vi "PicoScope2000ExampleStreaming.vi"() -> ()   [LabVIEW 2010]
doc: "This example demonstrates how to use the PicoScope Labview library to stream data from a PicoScope 2000 Series Device"
uses:
  PicoScope2000Lib/PicoScope2000AnalogChannelSettings.ctl
panel:
  in  "Write to file":bool
  in  "Trigger Settings":T1={"Trigger Enabled"=FALSE, "Trigger Source"=enum."Channel A", "Trigger Threshold (V)"=0.0, "Trigger Direction"=0, "Trigger Delay (%)"=-50, "Auto Trigger Time (ms)"=1000} {"Trigger Direction" items=["Rising", "Falling"]; "Trigger Threshold (V)" format="%.3p"}
  out "overflow":i16 format="%02b"
  out "Unit Info":T2
  out "Channels App Buffer":cluster{i32, dbl, "Channel B Buffer":i16[]}[](graph)
  in  "AutoStop App Buffer":bool
  in  "Channel A Settings":T3={"Enabled"=TRUE, "Coupling"=1, "Range"=6} {"Range" items=["20 mV"=1, "50 mV"=2, "100 mV"=3, "200 mV"=4, "500 mV"=5, "1 V"=6, "2 V"=7, "5 V"=8, "10 V"=9, "20 V"=10]; "Coupling" items=["AC", "DC"]}
  in  "Channel B Settings":T3={"Enabled"=TRUE, "Coupling"=1, "Range"=6} {"Range" items=["20 mV"=1, "50 mV"=2, "100 mV"=3, "200 mV"=4, "500 mV"=5, "1 V"=6, "2 V"=7, "5 V"=8, "10 V"=9, "20 V"=10]; "Coupling" items=["AC", "DC"]}
  out "Application Buffer Full":bool
  in  "Acquisition Settings":T4={"Auto Stop"=FALSE, "Desired Sample Interval"=2, "Max Samples"=333000, "Num Samples per Aggregate"=1, "Overview Buffer Size"=1000000, "Time Units"=3, "Application Buffer Size"=0} {"Time Units" items=["Nanoseconds (ns)"=2, "Microseconds (us)"=3, "Milliseconds (ms)"=4, "Seconds (s)"=5]; "Overview Buffer Size" format="%#.5p"; "Max Samples" format="%#.5p"}
  out "Analog Channels":T5(graph)
  out "Raw Sample Interval (sec)":dbl format="%#.5p"
  out "Chunk time":u32
  out "Elapsed time":dbl
  in  "Data file":path=path "PicoScope2000ExampleStreaming Data"
  out "Queue depth ChA":i32(graph)
  out "queue depth":i32
  in  "Buffer and Transfer Settings":T6={"startIndex"=0, "Samples"=1500000, "Down Sample Ratio"=1, "Down-Sample Mode"=0} {"Down-Sample Mode" items=["None"=0, "Aggregate"=1, "Decimate"=2, "Average"=4]; "Down Sample Ratio" step=1; "Samples" format="%#_5p"}
  out "TriggeredAt (In Buffer)":u32 format="%#.6p"
  out "TriggeredAt (Total samples)":u32 format="%#.6p"
  out "Triggered":bool
  out "DownSample Interval (sec)":dbl format="%#.5p"
  out "Total Samples":u32 format="%#.6p"
  out "Auto Stopped":bool
  out "Number of Samples per Capture":u32 format="%#.6p"
  in  "Apply  Settings":bool
  in  "stop":bool
  # "Max. Recommended Settings\nSettings for 1 channels\nSample Interval 1 us\n\nSettings for 2 channels\nSample Interval 2 us\n\nRecommended Settings-\nMax. Samples 333k\nOverview Buffer 1M\n\nBuffer and Transfer Settings-\nSamples- 1.5M (as min.)\n(Buffer = x1.5 (min) Overview buffer)"
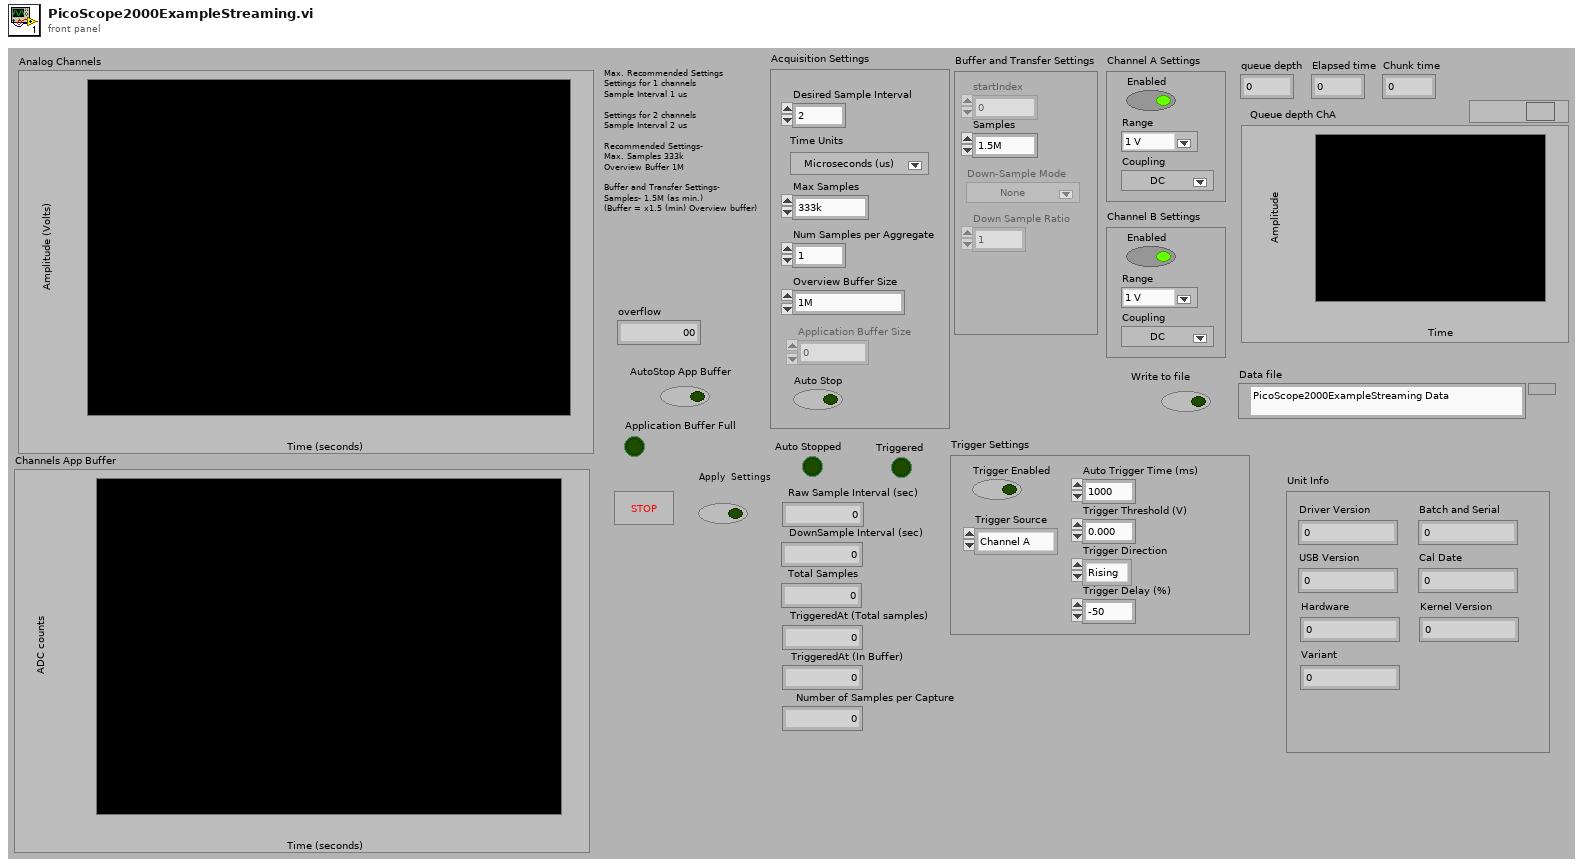
[diagram p1: front panel]
types:
  T1 = cluster{"Trigger Enabled":bool, "Trigger Source":enum16{"Channel A", "Channel B"}, "Trigger Threshold (V)":dbl, "Trigger Direction":i16, "Trigger Delay (%)":i16, "Auto Trigger Time (ms)":i16}
  T2 = cluster{"Driver Version":string, "USB Version":string, "Hardware":string, "Variant":string, "Batch and Serial":string, "Cal Date":string, "Kernel Version":string}
  T3 = typedef "PicoScope2000AnalogChannelSettings.ctl" = cluster{"Enabled":bool, "Coupling":i16, "Range":u16}
  T4 = cluster{"Auto Stop":bool, "Desired Sample Interval":u32, "Max Samples":u32, "Num Samples per Aggregate":u32, "Overview Buffer Size":u32, "Time Units":u32, "Application Buffer Size":u32}
  T5 = cluster{i32, "DownSample Interval (sec)":dbl, "Data":dbl[]}[]
  T6 = cluster{"startIndex":u64, "Samples":u64, "Down Sample Ratio":u64, "Down-Sample Mode":u32}
  T7 = enum16{"open", "open or create", "create or replace", "create", "open (read-only)"}
  T8 = cluster{"Channel A Buffer":i16[], "Channel B Buffer":i16[], "Channel C Buffer":i16[], "Channel D Buffer":i16[], "Channel E Buffer":i16[], "Channel F Buffer":i16[], "Channel G Buffer":i16[], "Channel H Buffer":i16[], "Port 0":i16[], "Port 1":i16[]}
  T9 = cluster{i32, "DownSample Interval (sec)":dbl, "Data":dbl[]}
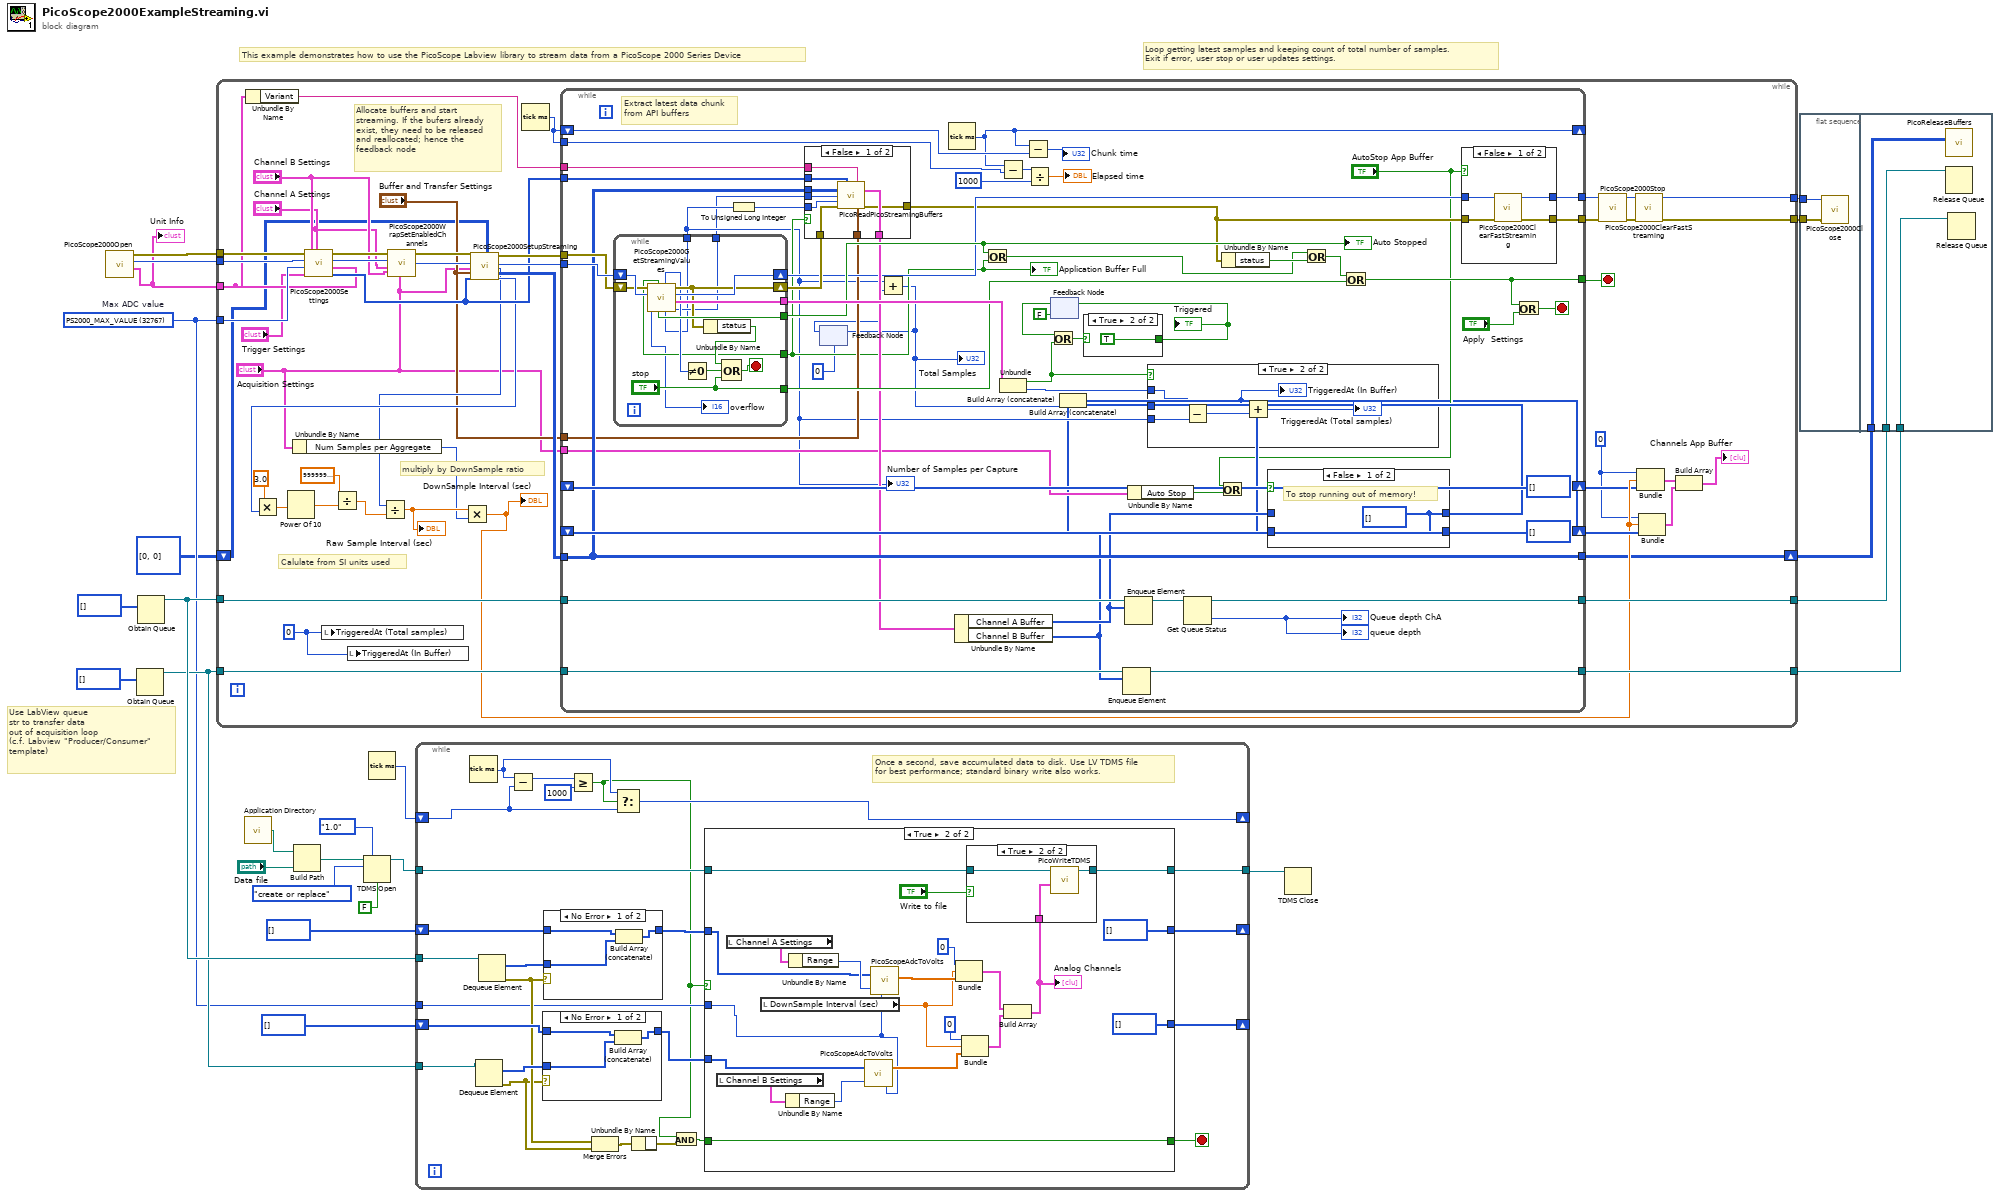
[diagram p0: block diagram]
diagram:
  w4 = i16 32767 items=["PS2000_MAX_VALUE"=32767]  # Max ADC value
  # "Loop getting latest samples and keeping count of total number of samples. \nExit if error, user stop or user updates settings."
  # "Use LabView queue\nstr to transfer data\nout of acquisition loop\n(c.f. Labview \"Producer/Consumer\"\ntemplate)"
  # "This example demonstrates how to use the PicoScope Labview library to stream data from a PicoScope 2000 Series Device"
  n1 = call "PicoScope2000Open.vi"() -> ("Unit Info"=w3:T2, "handle"=w24:i16, "error out"=w25:errorcluster)  [unwired: 7 in]
  "Unit Info" <- w3
  n2 = Obtain Queue(element data type=i16[] [] ("History Data")) -> (queue out=w5:refnum<queue>)  [unwired: 4 in, 2 out]
  n3 = Obtain Queue(element data type=i16[] [] ("History Data")) -> (queue out=w23:refnum<queue>)  [unwired: 4 in, 2 out]
  n4 = while {
    tunnel: [w47] -> w22
    tunnel: w25 -> [w74]
    tunnel: w24 -> [w75]
    tunnel: w3 -> [w60]
    tunnel: w4 -> [w64]
    tunnel: [w67] -> w21
    tunnel: w23 -> [w66]
    tunnel: [w48] -> w9
    tunnel: w5 -> [w56]
    tunnel: [w55] -> w7
    shift-right: [w32] -> w1
    shift-left: u64[][] [[0], [0]] ("Pointer array") -> [w33]
    stop <- w76 stop-if-true
    w28 = u32 0 ("TriggeredAt (Total samples)")
    w29 = 0
    # "multiply by DownSample ratio"
    # "Calulate from SI units used"
    # "Allocate buffers and start\nstreaming. If the bufers already\nexist, they need to be released\nand reallocated; hence the\nfeedback node"
    n5 = Unbundle By Name(w60) -> ("Variant"=w59:string)
    n6 = Unbundle By Name("Acquisition Settings") -> ("Num Samples per Aggregate"=w37:u32)
    n7 = call "PicoScope2000Settings.vi"("Unit Info"=w60, "Channel B Settings"="Channel B Settings", "Channel A Settings"="Channel A Settings", "Trigger Settings"="Trigger Settings", "Max ADC value"=w64, "handle in"=w75, "error in"=w74) -> ("Enabled Array"=w63:i16[], "handle out"=w68:i16, "error out"=w69:errorcluster)
    n8 = local write "TriggeredAt (Total samples)"(w28) -> ()
    n9 = local write "TriggeredAt (In Buffer)"(w28) -> ()
    n10 = call "PicoScope2000WrapSetEnabledChannels.vi"("Acquisition Settings"="Acquisition Settings", "Channel B Settings"="Channel B Settings", "Channel A Settings"="Channel A Settings", "handle in"=w68, "error in (no error)"=w69) -> ("handle out"=w71:i16, "error out"=w70:errorcluster)  [unwired: 1 in]
    n11 = call "PicoScope2000SetupStreaming.vi"("error in"=w70, "handle in"=w71, "Acquisition Settings"="Acquisition Settings", "Buffer and Transfer Settings"="Buffer and Transfer Settings", "enabled array"=w63, "Pointers In"=w33) -> ("Pointer array"=w65:u64[][], "error out"=w72:errorcluster, "handle out"=w73:i16, "Sample Interval"=w40:u32, "sampleIntervalTimeUnits"=w42:u32)  [unwired: 9 in]
    n12 = Multiply(x=3.0, y=w42) -> (x*y=w45:dbl)
    n13 = Power Of 10(x=w45) -> (10^x=w41:dbl)
    n14 = Divide(x=sgl 1000000000000000.0 ("y"), y=w41) -> (x/y=w39:dbl)
    n15 = Divide(x=w40, y=w39) -> (x/y=w38:dbl)
    "Raw Sample Interval (sec)" <- w38
    n16 = Multiply(x=w38, y=w37) -> (x*y=w35:dbl)
    "DownSample Interval (sec)" <- w35
    n17 = Tick Count (ms)() -> (millisecond timer value=w46:u32)
    n18 = while {
      tunnel: [w103] -> w58
      tunnel: [w134] -> w76
      tunnel: w73 -> [w124]
      tunnel: w72 -> [w123]
      tunnel: [w102] -> w57
      tunnel: "Buffer and Transfer Settings" -> [w100]
      tunnel: w63 -> [w121]
      tunnel: [w119] -> w67
      tunnel: w66 -> [w117]
      tunnel: w65 -> [w116]
      tunnel: [w116] -> w32
      shift-right: [w111] -> _
      shift-left: w46 -> [w112]
      tunnel: w59 -> [w109]
      tunnel: w56 -> [w97]
      tunnel: [w96] -> w55
      tunnel: w46 -> [w95]
      tunnel: "Acquisition Settings" -> [w93]
      shift-right: [w79] -> w30
      shift-left: i16[] [] ("Channel A Buffer") -> [w80]
      shift-right: [w77] -> w51
      shift-left: i16[] [] ("Channel B Buffer") -> [w78]
      stop <- w133 stop-if-true
      # "Extract latest data chunk\nfrom API buffers"
      n19 = while {
        tunnel: [w169] -> w132
        tunnel: [w168] -> w107
        tunnel: [w157] -> w81
        tunnel: [w156] -> w83
        shift-right: [w165] -> w104
        shift-left: w124 -> [w167]
        shift-right: [w164] -> w122
        shift-left: w123 -> [w166]
        tunnel: ["stop"] -> w108
        tunnel: [w158] -> w98
        stop <- w160 stop-if-true
        n20 = call "PicoScope2000GetStreamingValues.vi"("handle in"=w167, "error in"=w166) -> ("App Buffer startIndex"=w157:u32, "Trigger"=w169:cluster{bool, "triggeredAt  Index (Total)":u32}, "handle out"=w165:i16, "error out"=w164:errorcluster, "Number of Samples"=w156:u32, "ready"=w163:i16, "Auto Stopped"=w168:bool, "Application Buffer Full"=w158:bool, "overflow"=→"overflow":i16)  [unwired: 1 out]
        n21 = Not Equal To 0?(x=w163) -> (x != 0?=w161:bool)
        n22 = Unbundle By Name(w164) -> ("status"=w162:bool)
        n23 = Compound Arithmetic op=OR(w162, w161, "stop") -> (w160:bool)
      }
      "Number of Samples per Capture" <- w83
      "Auto Stopped" <- w107
      "Application Buffer Full" <- w98
      n24 = To Unsigned Long Integer(number=w83) -> (unsigned 32bit integer=w99:u32)
      n25 = case shown="False" w98 {
        tunnel: w122 -> [w153 w154]
        tunnel: w121 -> [w152 _]
        tunnel: w116 -> [w151 _]
        tunnel: w109 -> [w150 _]
        tunnel: [w149 _] -> w105
        tunnel: [w148 w154] -> w101
        tunnel: w100 -> [w147 _]
        tunnel: w99 -> [w146 _]
        tunnel: w81 -> [w145 _]
        frame False {
          n26 = call "PicoReadPicoStreamingBuffers.vi"("enabled array"=w152, "Buffer and Transfer Settings"=w147, "Variant"=w150, "Pointer array"=w151, "Offset Index"=w145, "Number of Samples"=w146, "error in (no error)"=w153) -> ("Buffers (Max or non-aggregated)"=w149:T8, "error out"=w148:errorcluster)  [unwired: 6 in, 1 out]
        }
        frame True {
        }
      }
      n27 = feedback #1(u32 0) -> (w85:u32)
      n28 = Add(x=w83, y=w85) -> (x+y=w82:u32)
      "Total Samples" <- w82
      n29 = feedback-in #1(w82) -> ()
      n30 = Tick Count (ms)() -> (millisecond timer value=w111:u32)
      n31 = Unbundle By Name(w105) -> ("Channel A Buffer"=w92:i16[], "Channel B Buffer"=w91:i16[])
      n32 = Or(x=w107, y=w98) -> (x .or. y?=w106:bool)
      n33 = Subtract(x=w111, y=w95) -> (x-y=w115:u32)
      n34 = Unbundle(w132) -> (w86:bool, "triggeredAt  Index (Total)"=w125:u32)
      n35 = Subtract(x=w111, y=w112) -> (x-y=→"Chunk time":u32)
      n36 = Divide(x=w115, y=u32 1000) -> (x/y=→"Elapsed time":dbl)
      n37 = feedback #2(FALSE) -> (w129:bool)
      n38 = Or(x=w129, y=w86) -> (x .or. y?=w127:bool)
      n39 = case shown="True" w127 {
        selector: w127 -> [w175 _]
        tunnel: [w175 TRUE] -> w126
        frame False {
        }
        frame True {
        }
      }
      "Triggered" <- w126
      n40 = feedback-in #2(w126) -> ()
      n41 = Enqueue Element(queue=w97, element=w91) -> (queue out=w96:refnum<queue>)  [unwired: 2 in, 2 out]
      n42 = Enqueue Element(queue=w117, element=w92) -> (queue out=w118:refnum<queue>)  [unwired: 2 in, 2 out]
      n43 = Unbundle By Name(w93) -> ("Auto Stop"=w89:bool)
      n44 = case shown="True" w86 {
        tunnel: w83 -> [_ w171]
        tunnel: w82 -> [_ w174]
        tunnel: w125 -> [_ w170]
        frame False {
        }
        frame True {
          n45 = Subtract(x=w174, y=w171) -> (x-y=w173:u32)
          n46 = Add(x=w170, y=w173) -> (x+y=→"TriggeredAt (Total samples)":u32)
          "TriggeredAt (In Buffer)" <- w170
        }
      }
      n47 = Get Queue Status(queue=w118) -> (queue out=w119:refnum<queue>, # elements in queue=→"queue depth" →"Queue depth ChA":i32)  [unwired: 2 in, 6 out]
      n48 = Or(x="AutoStop App Buffer", y=w89) -> (x .or. y?=w88:bool)
      n49 = Unbundle By Name(w101) -> ("status"=w131:bool)
      n50 = case shown="False" w88 {
        tunnel: [w136 w138] -> w94
        tunnel: w92 -> [_ w138]
        tunnel: w91 -> [_ w137]
        tunnel: [w136 w137] -> w90
        frame False {
          w136 = i16[] [] ("Channel A Buffer")
          # "To stop running out of memory!"
        }
        frame True {
        }
      }
      n51 = Build Array (concatenate)(w78, w90) -> (w77:i16[])
      n52 = Build Array (concatenate)(w80, w94) -> (w79:i16[])
      n53 = Or(x=w106, y=w131) -> (x .or. y?=w130:bool)
      n54 = Or(x=w130, y=w108) -> (x .or. y?=w134:bool)
      n55 = case shown="False" "AutoStop App Buffer" {
        tunnel: w104 -> [w142 w143]
        tunnel: [w139 w143] -> w103
        tunnel: [w140 w144] -> w102
        tunnel: w101 -> [w141 w144]
        frame False {
          n56 = call "PicoScope2000ClearFastStreaming.vi"("error in"=w141, "handle"=w142) -> ("error out"=w140:errorcluster, "handle out"=w139:i16)  [unwired: 4 in]
        }
        frame True {
        }
      }
      n57 = Or(x=w134, y="Apply  Settings") -> (x .or. y?=w133:bool)
    }
    n58 = call "PicoScope2000Stop.vi"("error in (no error)"=w57, "handle in"=w58) -> ("error out"=w50:errorcluster, "handle out"=w49:i16)  [unwired: 8 in]
    n59 = call "PicoScope2000ClearFastStreaming.vi"("error in"=w50, "handle"=w49) -> ("error out"=w48:errorcluster, "handle out"=w47:i16)  [unwired: 4 in]
    n60 = Bundle(w29, w35, "Channel A Buffer"=w30) -> (w54:cluster{i32, dbl, "Channel A Buffer":i16[]})  [unwired: 1 in]
    n61 = Bundle(w29, w35, "Channel B Buffer"=w51) -> (w53:cluster{i32, dbl, "Channel B Buffer":i16[]})  [unwired: 1 in]
    n62 = Build Array(w54, w53) -> (→"Channels App Buffer":cluster{i32, dbl, "Channel B Buffer":i16[]}[])
  }
  n63 = call <vilib>:"Application Directory.vi"() -> ("Application Directory"=w10:path)
  n64 = Build Path(base path=w10, name or relative path="Data file") -> (appended path=w11:path)
  n65 = TDMS Open(6:FALSE ("disable buffering? (T)"), 7:enum16{"1.0", "2.0"}."1.0" ("file format version (2.0)"), 10:T7."create or replace" ("operation (0:open)"), 11:w11) -> (3:w18:refnum<k34>)  [unwired: 2 in, 1 out]
  n66 = Tick Count (ms)() -> (millisecond timer value=w20:u32)
  n67 = while {
    tunnel: w23 -> [w200]
    shift-right: [w192] -> _
    shift-left: i16[] [] ("History Data") -> [w199]
    shift-right: [w194] -> _
    shift-left: w20 -> [w195]
    tunnel: w18 -> [w191]
    tunnel: [w190] -> w17
    tunnel: w5 -> [w189]
    shift-right: [w185] -> _
    shift-left: i16[] [] ("History Data") -> [w188]
    tunnel: w4 -> [w181]
    stop <- w182 stop-if-true
    # "Once a second, save accumulated data to disk. Use LV TDMS file\nfor best performance; standard binary write also works."
    n68 = Tick Count (ms)() -> (millisecond timer value=w196:u32)
    n69 = Dequeue Element(queue=w189) -> (element=w187:i16[], error out=w183:errorcluster)  [unwired: 2 in, 2 out]
    n70 = Dequeue Element(queue=w200) -> (element=w201:i16[], error out=w184:errorcluster)  [unwired: 2 in, 2 out]
    n71 = Subtract(x=w196, y=w195) -> (x-y=w198:u32)
    n72 = case shown="No Error" w183 {
      tunnel: w188 -> [w204 w205]
      tunnel: [w203 w205] -> w186
      tunnel: w187 -> [w202 _]
      frame No Error {
        n73 = Build Array (concatenate)(w204, w202) -> (w203:i16[])
      }
      frame Error {
      }
    }
    n74 = case shown="No Error" w184 {
      tunnel: w199 -> [w237 w238]
      tunnel: [w236 w238] -> w193
      tunnel: w201 -> [w235 _]
      frame No Error {
        n75 = Build Array (concatenate)(w237, w235) -> (w236:i16[])
      }
      frame Error {
      }
    }
    n76 = Greater Or Equal?(x=w198, y=u32 1000) -> (x >= y?=w178:bool)
    n77 = Merge Errors(w184, w183) -> (w180:errorcluster)
    n78 = Select(t=w196, s=w178, f=w195) -> (s? t:f=w194:u32)
    n79 = And(x=w178) -> (y=w177:errorcluster, x .and. y?=w179:bool)
    n80 = Unbundle By Name(w180, w177) -> ()
    n81 = case shown="True" w178 {
      tunnel: w193 -> [w209 w212]
      tunnel: [w209 i16[] [] ("History Data")] -> w192
      tunnel: w191 -> [w208 w229]
      tunnel: [w208 w228] -> w190
      tunnel: w186 -> [w207 w217]
      tunnel: [w207 i16[] [] ("History Data")] -> w185
      tunnel: [w206 w214] -> w182
      tunnel: w179 -> [w206 w214]
      tunnel: w181 -> [_ w213]
      frame False {
      }
      frame True {
        n82 = local read "Channel B Settings"() -> (w216:T3)
        n83 = local read "Channel A Settings"() -> (w224:T3)
        n84 = local read "DownSample Interval (sec)"() -> (w220:dbl)
        n85 = Unbundle By Name(w216) -> ("Range"=w218:u16)
        n86 = Unbundle By Name(w224) -> ("Range"=w227:u16)
        n87 = call "PicoScopeAdcToVolts.vi"("Max_adc"=w213, "Range Index"=w218, "Data"=w217) -> ("Data"=w219:dbl[])
        n88 = call "PicoScopeAdcToVolts.vi"("Max_adc"=w213, "Range Index"=w227, "Data"=w212) -> ("Data"=w225:dbl[])
        n89 = Bundle(0, "DownSample Interval (sec)"=w220, "Data"=w225) -> (w223:T9)  [unwired: 1 in]
        n90 = Bundle(0, "DownSample Interval (sec)"=w220, "Data"=w219) -> (w222:T9)  [unwired: 1 in]
        n91 = Build Array(w223, w222) -> (w210:T5)
        "Analog Channels" <- w210
        n92 = case shown="True" "Write to file" {
          tunnel: w229 -> [w231 w233]
          tunnel: [w231 w234] -> w228
          tunnel: w210 -> [_ w232]
          frame False {
          }
          frame True {
            n93 = call "PicoWriteTDMS.vi"("Analog Channels"=w232, "Refnum in"=w233) -> ("Refnum out"=w234:refnum<k34>)  [unwired: 8 in, 1 out]
          }
        }
      }
    }
  }
  n94 = TDMS Close(11:w17) -> ()  [unwired: 1 in, 2 out]
  n95 = flat-sequence {
    tunnel: w22 -> [w240]
    tunnel: w9 -> [w239]
    tunnel: w1 -> [w243]
    tunnel: w21 -> [w242]
    tunnel: w7 -> [w241]
    frame #0 {
      n96 = call "PicoScope2000Close.vi"("error in"=w239, "handle"=w240) -> ()  [unwired: 4 in, 2 out]
    }
    frame #1 {
      n97 = call "PicoReleaseBuffers.vi"("Pointer array"=w243) -> ()  [unwired: 9 in, 2 out]
      n98 = Release Queue(queue=w242) -> ()  [unwired: 2 in, 3 out]
      n99 = Release Queue(queue=w241) -> ()  [unwired: 2 in, 3 out]
    }
  }
